vi "Save Table Test for NG.vi"(8 "error in (no error)":errorcluster, 11 "SN":string) -> (0 "error out":errorcluster, 3 "條碼的Index":i32)   [LabVIEW 2019]
uses:
  Ctrl/Table Save.ctl
  LLB/Message/Ctrl/LogType.ctl
  <vilib>/Utility/sysdir.llb/System Directory Type.ctl
  <vilib>/Utility/file.llb/Write Delimited Spreadsheet (string).vi
  LLB/Message/MsgShowAndLog.lvlib
panel:
  out "Read SN Table":string[][](array[string])
  in  "Base Path":path=path "D:/Vicomm"
  out "element":string
  in  "Cluster":cluster{"Table Control":string[][]}={"Table Control"=[["PCBA BARCODE", ""], ["硬體(Tool初始化)", ""], ["company(Tool初始化)", ""], ["耗電流 uA(電流表)", "T"], ["電池負載電壓", "T"], ["晶片ID(Tool FORMAT)", "F"], ["雷雕ID(TOOl scan、藍芽接收器)", "S"], ["Format(Tool FORMAT)", "F"], ["Programe(Tool Programe)", "P"]]}
  # "-1 : 未找到條碼"
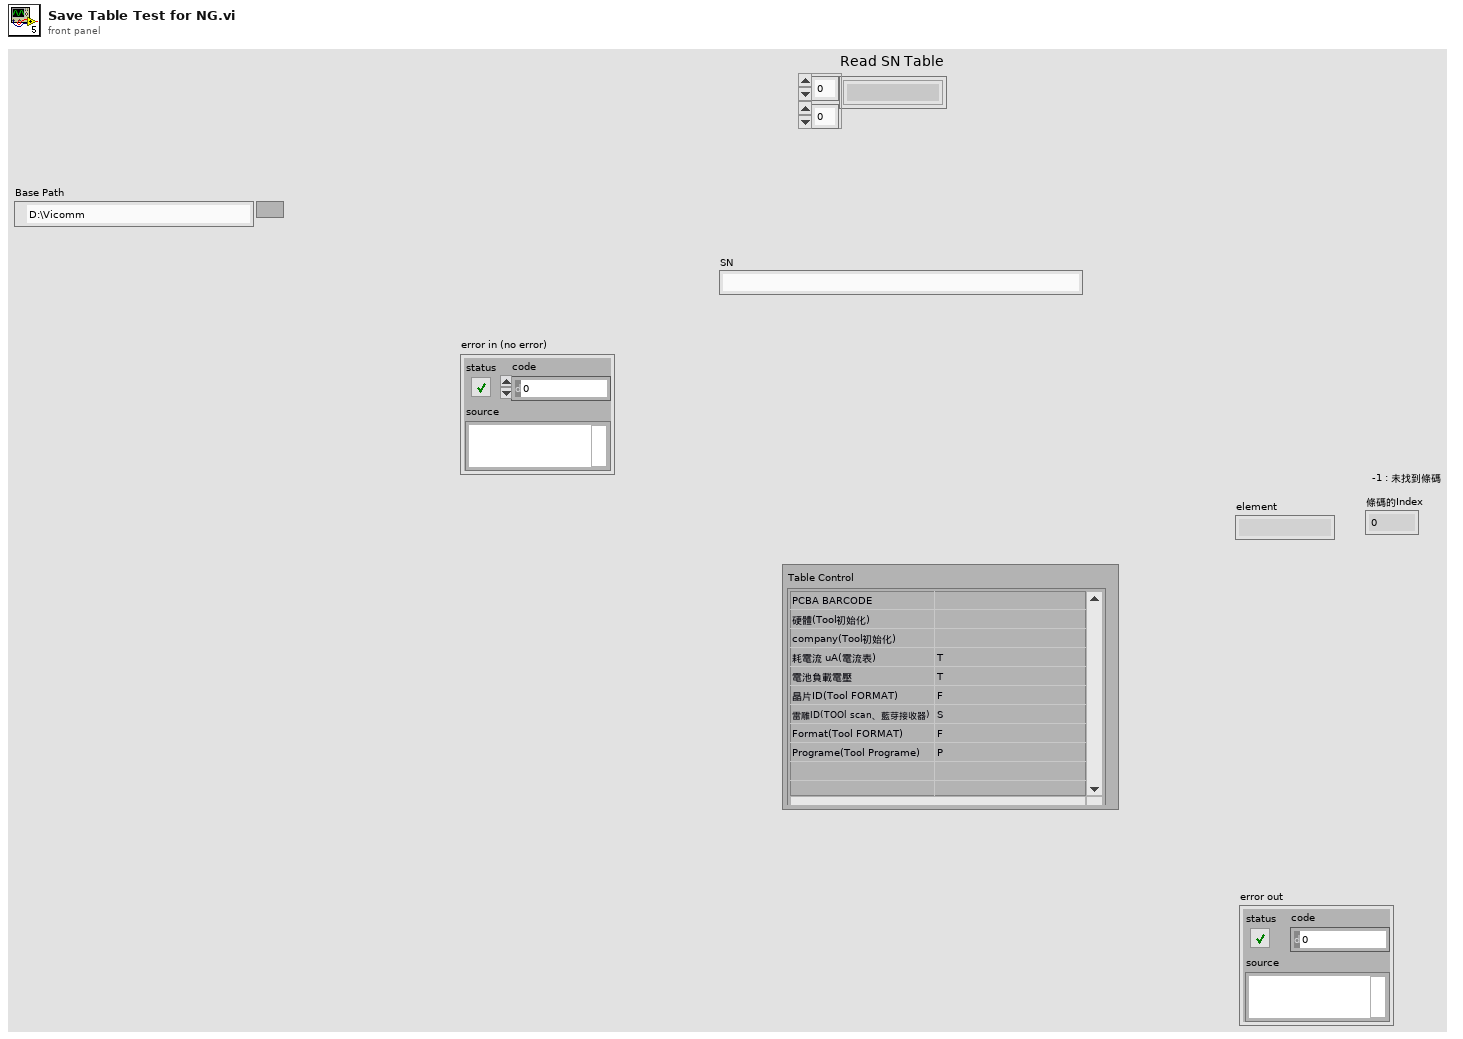
[diagram p1: front panel]
types:
  T1 = typedef "Table Save.ctl" = enum16{"initial", "Add", "Write", "Replace", "Delete", "REad", "RedTable", "Load"}
  T2 = enum16{"open", "replace", "create", "open or create", "replace or create", "replace or create with confirmation"}
  T3 = typedef "MsgShowAndLog.lvlib/LogType.ctl" = enum16{"Auto", "Manual", "Handshake", "Error"}
  T4 = typedef "System Directory Type.ctl" = i32
  T5 = typedef "LVDateTimeRec.ctl" = cluster{"fractional second":dbl, "second":i32, "minute":i32, "hour":i32, "day of month":i32, "month":i32, "year":i32, "day of week":i32, "day of year":i32, "DST":i32}
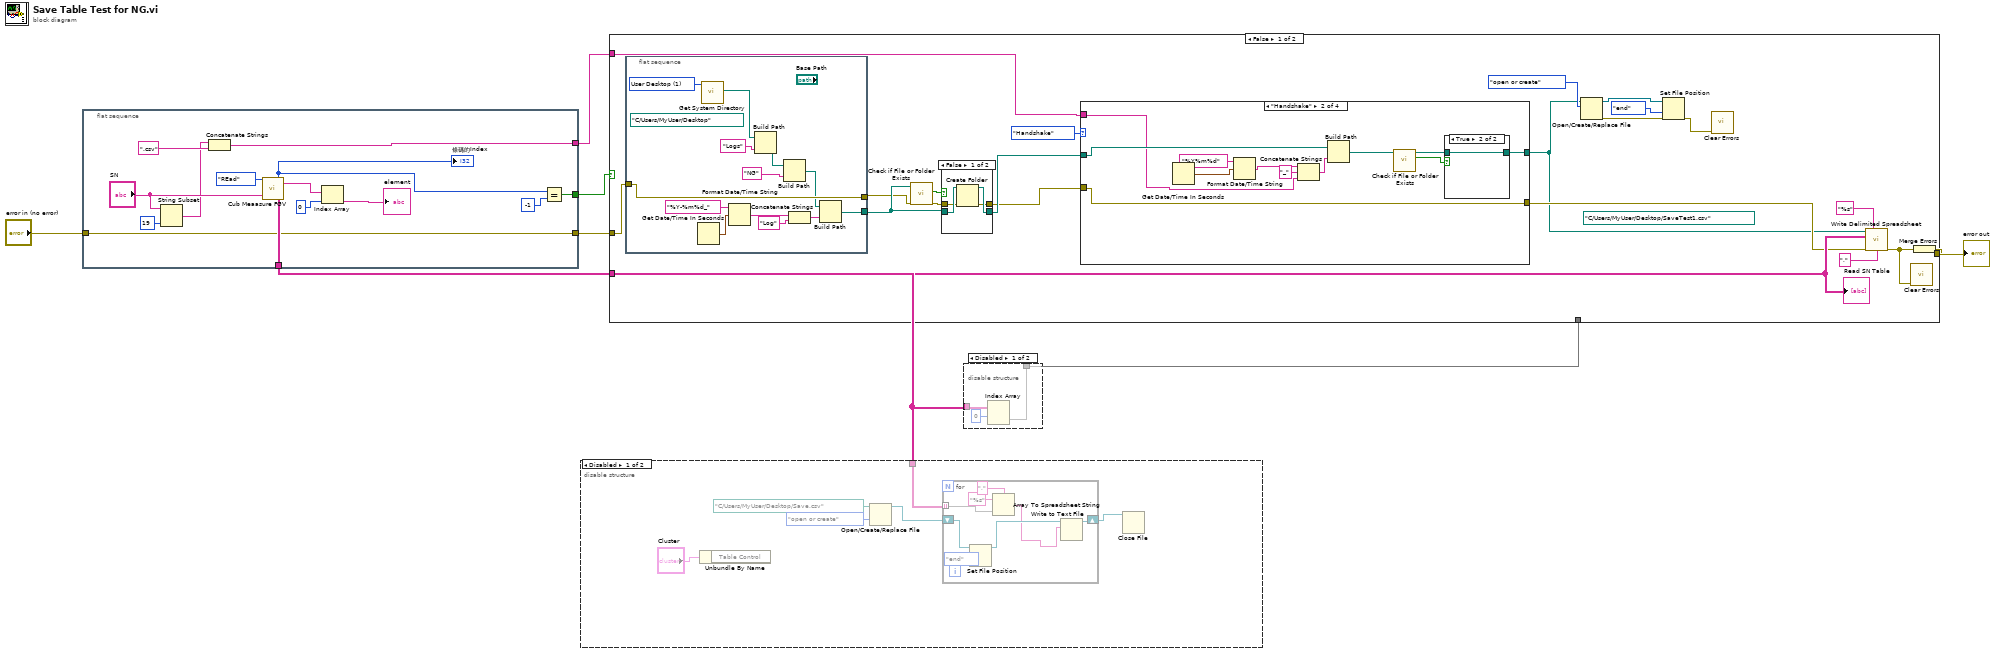
[diagram p0: block diagram]
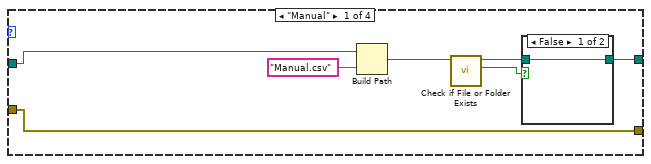
[diagram p2: hidden frame]
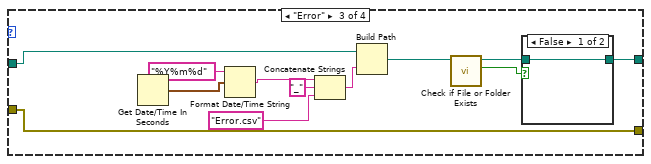
[diagram p5: hidden frame]
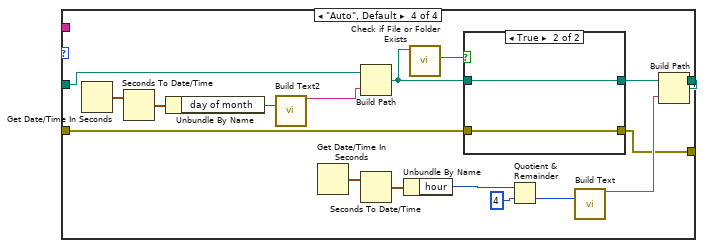
[diagram p7: hidden frame]
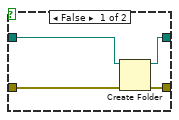
[diagram p8: hidden frame]
diagram:
  n1 = flat-sequence {
    tunnel: [w21] -> w1
    tunnel: [w15] -> w6
    tunnel: "error in (no error)" -> [w12]
    tunnel: [w12] -> w3
    tunnel: [w11] -> w4
    frame #0 {
      n2 = String Subset(string="SN", length (rest)=19 ("length (rest)")) -> (substring=w9:string)  [unwired: 1 in]
      n3 = Concatenate Strings(w9, ".csv") -> (w21:string)
      n4 = call "Cub Meaasure FGV.vi"("Action"=Table_Save."REad", "SN"="SN") -> ("條碼的Index"=w14:i32, "Read SN Table"=w15:string[][], "Barcode Array"=w17:string[])  [unwired: 10 in, 5 out]
      "條碼的Index" <- w14
      n5 = Index Array(array=w17, index=0) -> (element=→"element":string)
      n6 = Equal?(x=w14, y=-1) -> (x = y?=w11:bool)
    }
  }
  n7 = disable-structure shown="Disabled" {
    disable-tunnel: w6 -> [w23 _]
    frame Disabled {
      n8 = Unbundle By Name("Cluster") -> ()  [unwired: 1 out]
      n9 = Open/Create/Replace File(file path (use dialog)=path "C:/Users/MyUser/Desktop/Save.csv", operation (0:open)=T2."open or create") -> (refnum out=w27:refnum<file>)  [unwired: 4 in, 2 out]
      n10 = for {
        tunnel: w23 -> [w35] mode=indexing
        shift-right: [w32] -> w25
        shift-left: w27 -> [w31]
        n11 = Set File Position(refnum=w31, from (0:start)=enum16{"start", "end", "current"}."end") -> (refnum out=w30:refnum<file>)  [unwired: 2 in, 1 out]
        n12 = Array To Spreadsheet String(delimiter (Tab)=",", array=w35, 3:"%s" ("format string")) -> (spreadsheet string=w28:string)
        n13 = Write to Text File(file (use dialog)=w30, text=w28) -> (refnum out=w32:refnum<file>)  [unwired: 2 in, 2 out]
      }
      n14 = Close File(refnum=w25) -> ()  [unwired: 1 in, 2 out]
    }
    frame Enabled {
    }
  }
  n15 = disable-structure shown="Disabled" {
    disable-tunnel: [w37 _] -> w7
    disable-tunnel: w6 -> [w36 _]
    frame Disabled {
      n16 = Index Array(array=w36, index (row)=0) -> (element=w37:string[])  [unwired: 1 in]
    }
    frame Enabled {
    }
  }
  n17 = case shown="False" w4 {
    tunnel: w7 -> [_ _]
    tunnel: w6 -> [w48 _]
    tunnel: w3 -> [w42 w139]
    tunnel: [w41 w139] -> w2
    tunnel: w1 -> [w40 _]
    frame False {
      (unwired) path "C:/Users/MyUser/Desktop/SaveTest1.csv" ("file path (dialog if empty)")
      n18 = flat-sequence {
        tunnel: [w126] -> w58
        tunnel: w42 -> [w125]
        tunnel: [w125] -> w56
        frame #0 {
          w124 = T4 1 items=["User Home"=0, "User Desktop"=1, "User Documents"=2, "User Application Data"=3, "User Preferences"=4, "User Temporary"=5, "Public Documents"=6, "Public Application Data"=7, "Public Preferences"=8, "Public Cache"=13, "System Core Libraries"=9, "System Installed Libraries"=10, "Application Files"=11, "Boot Volume Root"=12] ("system directory type")
          (unwired) path "C:/Users/MyUser/Desktop" ("file path (dialog if empty)")
          n19 = Get Date/Time In Seconds() -> (seconds since 1Jan1904=w127:timestamp)
          n20 = call <vilib>:"Get System Directory.vi"("system directory type"=w124) -> ("system directory"=w123:path)  [unwired: 10 in]
          n21 = Format Date/Time String(time format string (%c)="%Y-%m%d_", seconds (now)=w127) -> (date/time string=w129:string)  [unwired: 1 in]
          n22 = Build Path(base path=w123, name or relative path="Logs") -> (appended path=w121:path)
          n23 = Build Path(base path=w121, name or relative path="NG") -> (appended path=w120:path)
          n24 = Concatenate Strings(w129, "Log") -> (w131:string)
          n25 = Build Path(base path=w120, name or relative path=w131) -> (appended path=w126:path)
        }
      }
      n26 = call <vilib>:"Check if File or Folder Exists.vi"("error in (no error)"=w56, "path"=w58) -> ("error out"=w59:errorcluster, "file or folder exists?"=w57:bool)  [unwired: 7 in, 1 out]
      n27 = case shown="False" w57 {
        tunnel: w58 -> [w136 w138]
        tunnel: [w135 w138] -> w54
        tunnel: w59 -> [w134 w137]
        tunnel: [w133 w137] -> w53
        frame False {
          n28 = Create Folder(path (use dialog)=w136, error in=w134) -> (created path=w135:path, error out=w133:errorcluster)  [unwired: 1 in, 1 out]
        }
        frame True {
        }
      }
      n29 = case shown="\"Handshake\"" LogType."Handshake" ("LogType") {
        tunnel: w54 -> [w66 w80 w94 w108]
        tunnel: w53 -> [w60 w75 w89 w101]
        tunnel: [w61 w76 w90 w100] -> w39
        tunnel: [w60 w75 w89 w97] -> w43
        tunnel: w40 -> [_ w69 _ _]
        frame "Manual" {
          n30 = Build Path(base path=w66, name or relative path="Manual.csv") -> (appended path=w64:path)
          n31 = call <vilib>:"Check if File or Folder Exists.vi"("path"=w64) -> ("file or folder exists?"=w63:bool, "dup path"=w62:path)  [unwired: 8 in, 1 out]
          n32 = case shown="False" w63 {
            tunnel: w62 -> [w67 w68]
            tunnel: [w67 w68] -> w61
            frame False {
            }
            frame True {
            }
          }
        }
        frame "Handshake" {
          n33 = Get Date/Time In Seconds() -> (seconds since 1Jan1904=w74:timestamp)
          n34 = Format Date/Time String(time format string (%c)="%Y%m%d", seconds (now)=w74) -> (date/time string=w71:string)  [unwired: 1 in]
          n35 = Concatenate Strings(w71, "_" ("string"), w69) -> (w72:string)
          n36 = Build Path(base path=w80, name or relative path=w72) -> (appended path=w79:path)
          n37 = call <vilib>:"Check if File or Folder Exists.vi"("path"=w79) -> ("file or folder exists?"=w78:bool, "dup path"=w77:path)  [unwired: 8 in, 1 out]
          n38 = case shown="True" w78 {
            tunnel: w77 -> [w81 w82]
            tunnel: [w81 w82] -> w76
            frame False {
            }
            frame True {
            }
          }
        }
        frame "Error" {
          n39 = Get Date/Time In Seconds() -> (seconds since 1Jan1904=w88:timestamp)
          n40 = Format Date/Time String(time format string (%c)="%Y%m%d", seconds (now)=w88) -> (date/time string=w84:string)  [unwired: 1 in]
          n41 = Concatenate Strings(w84, "_" ("string"), "Error.csv" ("name or relative path")) -> (w86:string)
          n42 = Build Path(base path=w94, name or relative path=w86) -> (appended path=w93:path)
          n43 = call <vilib>:"Check if File or Folder Exists.vi"("path"=w93) -> ("file or folder exists?"=w92:bool, "dup path"=w91:path)  [unwired: 8 in, 1 out]
          n44 = case shown="False" w92 {
            tunnel: w91 -> [w95 w96]
            tunnel: [w95 w96] -> w90
            frame False {
            }
            frame True {
            }
          }
        }
        frame "Auto", Default {
          n45 = Get Date/Time In Seconds() -> (seconds since 1Jan1904=w106:timestamp)
          n46 = Seconds To Date/Time(time stamp (now)=w106) -> (date time rec=w105:T5)  [unwired: 1 in]
          n47 = Unbundle By Name(w105) -> ("day of month"=w107:i32)
          n48 = call "Build Text2"("Date"=w107) -> ("Result"=w104:string)  [unwired: 13 in, 1 out]
          n49 = Get Date/Time In Seconds() -> (seconds since 1Jan1904=w113:timestamp)
          n50 = Build Path(base path=w108, name or relative path=w104) -> (appended path=w99:path)
          n51 = Seconds To Date/Time(time stamp (now)=w113) -> (date time rec=w112:T5)  [unwired: 1 in]
          n52 = Unbundle By Name(w112) -> ("hour"=w110:i32)
          n53 = call <vilib>:"Check if File or Folder Exists.vi"("path"=w99) -> ("file or folder exists?"=w98:bool)  [unwired: 8 in, 2 out]
          n54 = case shown="True" w98 {
            tunnel: w99 -> [w117 w119]
            tunnel: [w116 w119] -> w103
            tunnel: w101 -> [w115 w118]
            tunnel: [w114 w118] -> w97
            frame False {
              n55 = Create Folder(path (use dialog)=w117, error in=w115) -> (created path=w116:path, error out=w114:errorcluster)  [unwired: 1 in, 1 out]
            }
            frame True {
            }
          }
          n56 = Quotient & Remainder(x=w110, y=4) -> (floor(x/y)=w109:i32)  [unwired: 1 out]
          n57 = call "Build Text"("Time"=w109) -> ("Result"=w102:string)  [unwired: 13 in, 1 out]
          n58 = Build Path(base path=w103, name or relative path=w102) -> (appended path=w100:path)
        }
      }
      n59 = Open/Create/Replace File(file path (use dialog)=w39, operation (0:open)=T2."open or create") -> (refnum out=w50:refnum<file>, error out=w52:errorcluster)  [unwired: 4 in, 1 out]
      n60 = Set File Position(refnum=w50, from (0:start)=enum16{"start", "end", "current"}."end", error in=w52) -> (error out=w47:errorcluster)  [unwired: 1 in, 1 out]
      n61 = call <vilib>:"Clear Errors.vi"("error in (no error)"=w47) -> ()  [unwired: 5 in, 2 out]
      n62 = call-poly <vilib>:"Write Delimited Spreadsheet.vi"("file path (dialog if empty)"=w39, "format (%s)"="%s", "2D data"=w48, "error in (no error)"=w43, "delimiter (\\t)"="," ("delimiter (\\t)")) -> ("error out"=w44:errorcluster)  [unwired: 9 in, 1 out]
      n63 = call <vilib>:"Clear Errors.vi"("error in (no error)"=w44) -> ()  [unwired: 5 in, 2 out]
      n64 = Merge Errors(w44) -> (w41:errorcluster)
      "Read SN Table" <- w48
    }
    frame True {
    }
  }
  "error out" <- w2
